vi "Read Acquisition.vi"(8 "error in (no error)":errorcluster, 11 "Initialize_card in":refnum<class "Control_card.lvclass">) -> (0 "error out":errorcluster, 2 "Acquisition":T1={"Sample Rate"=10000000.0, "Clock mode"=enum."Internal", "Mode"=0, "Depth"=8160.0, "Segment Size"=8160.0, "Trigger Timeout"=1000000.0, "Trigger Holdoff"=0.0, "Trigger Delay"=0.0} {"Segment Size" min=160.0 step=160.0; "Trigger Holdoff" min=0.0 step=160.0; "Trigger Delay" min=0.0 step=160.0; "Depth" min=160.0 step=160.0; "Mode" items=["Single", "Dual", "Quad", "Octal"]}, 3 "Initialize_card out":refnum<class "Control_card.lvclass">)   [LabVIEW 2015, in "Control_card.lvclass"]
uses:
  Control_card.lvclass
  Control_card.lvclass/Control_card.ctl
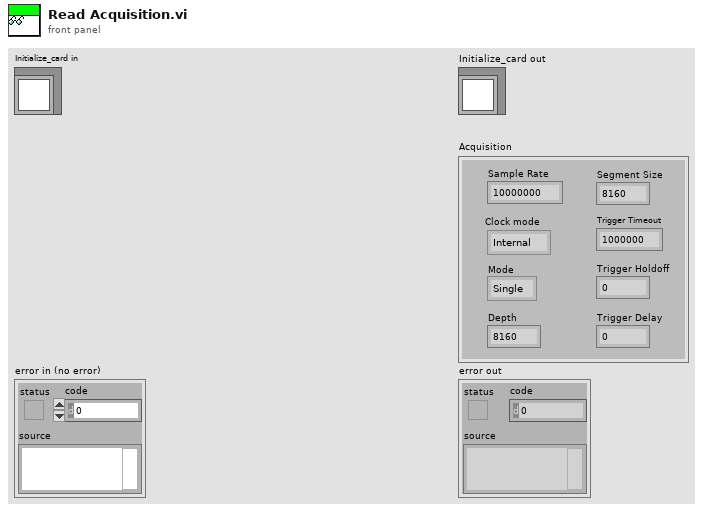
[diagram p1: front panel]
types:
  T1 = cluster{"Sample Rate":dbl, "Clock mode":enum16{"Internal", "External", "Reference"}, "Mode":u16, "Depth":dbl, "Segment Size":dbl, "Trigger Timeout":dbl, "Trigger Holdoff":dbl, "Trigger Delay":dbl}
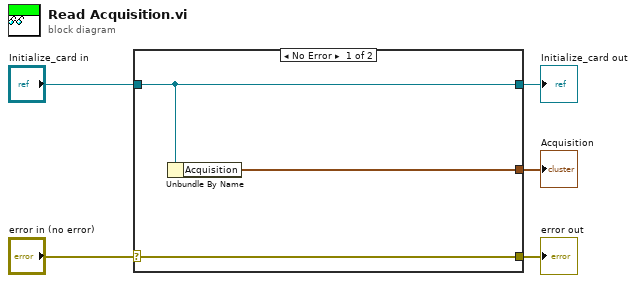
[diagram p0: block diagram]
diagram:
  n1 = case shown="No Error" "error in (no error)" {
    selector: "error in (no error)" -> [w8 w9]
    tunnel: [w8 w9] -> w4
    tunnel: [w7 w10] -> w2
    tunnel: "Initialize_card in" -> [w7 w10]
    tunnel: [w6 _] -> w1
    frame No Error {
      n2 = Unbundle By Name(w7) -> ("Acquisition"=w6:T1)
    }
    frame Error {
    }
  }
  "error out" <- w4
  "Initialize_card out" <- w2
  "Acquisition" <- w1
